vi "Extract_ROIs_miniScans.vi"(5 "ROI Attributes":T1[](array[typedef]) {"Apparent Frame Size" format="%#_6f"; "Original FOV (um)" format="%#_6f"; "Pixels per miniscan" format="%#_6f"; "Dwell Time per pixel" format="%#_6f"; "Resolution" format="%#_6f"; "ROI group ID" format="%#_6f"; "Laser Power (%)" format="%#_6f"; "Zoom" format="%#_6f"; "Frame Size" format="%#_6f"; "Number of lines" format="%#_6f"; "Composite ID" format="%#_6f"; "Angle (deg)" format="%#_6f"; "ROI Time (ns)" format="%#_6f"; "ROI ID" format="%#_6f"; "Pixels in ROI" format="%#_6f"; "ROI index" format="%#_6f"; "Z stop" format="%#_6f"; "Y stop" format="%#_6f"; "X stop" format="%#_6f"; "Z start" format="%#_6f"; "X start" format="%#_6f"; "Y start" format="%#_6f"}, 11 "error in (no error)":errorcluster) -> (1 "number of POI":i32, 3 "Number of pixels in single X miniscan":i32, 4 "ROI Coordinates (broken down to miniscans)":T2, 6 "miniScan_Indices":dbl[](array[numeric]), 8 "Total Pixels":i32, 10 "Total number of miniscans":i32, 12 "number of rectangles":i32, 13 "variable X Miniscan Pixels":i32[](array[numeric]), 14 "Zoom":dbl[](array[numeric]), 15 "error out":errorcluster)   [LabVIEW 2020]
uses:
  Typedefs/ROI XY coordinates cluster.ctl
  User Interface/Visualisation/Functional Imaging Viewer/Typedefs/ROI parameters data type.ctl
panel:
  out "POI_Indices":dbl[](array[numeric])
  # "PRE-ALLOCATED CLONE RE-ENTRANT"
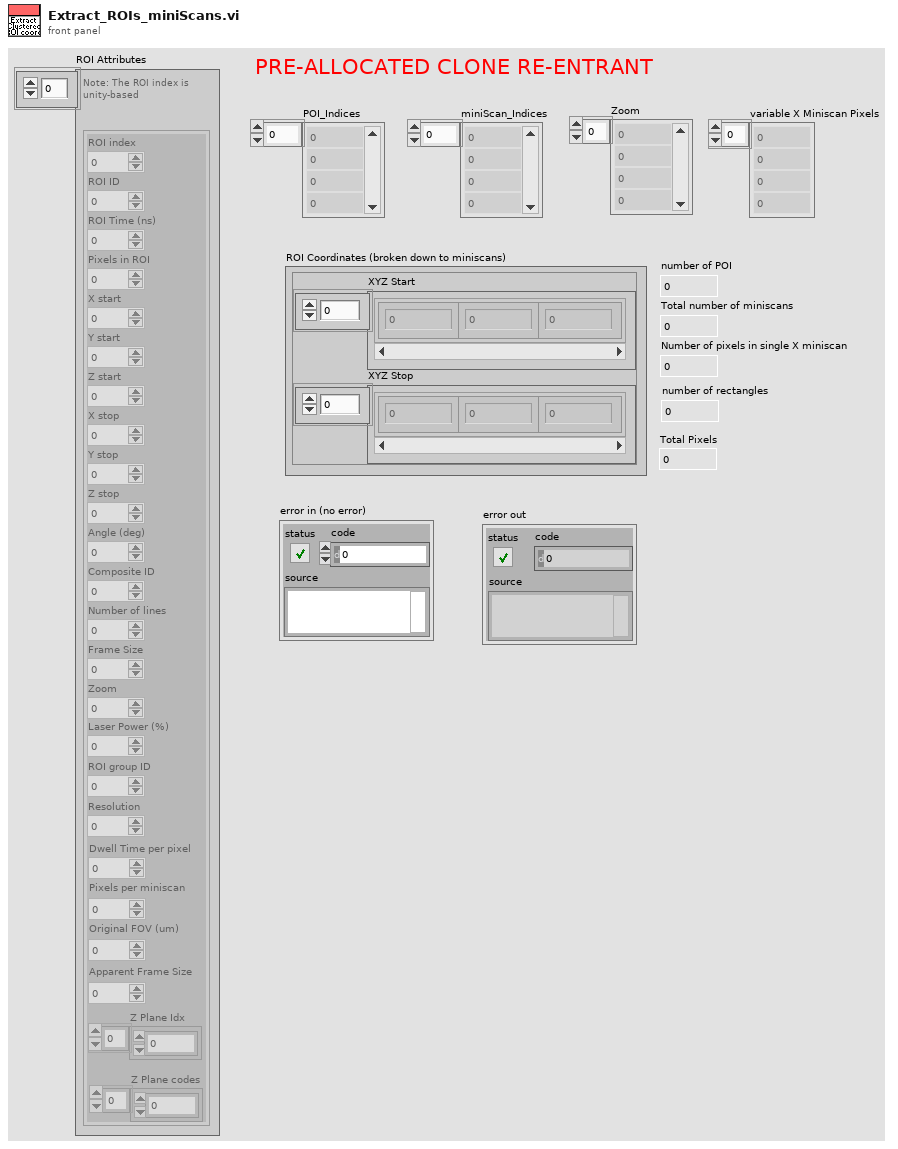
[diagram p1: front panel]
types:
  T1 = typedef "ROI parameters data type.ctl" = cluster{"ROI index":dbl, "ROI ID":dbl, "ROI Time (ns)":dbl, "Pixels in ROI":dbl, "X start":dbl, "Y start":dbl, "Z start":dbl, "X stop":dbl, "Y stop":dbl, "Z stop":dbl, "Angle (deg)":dbl, "Composite ID":dbl, "Number of lines":dbl, "Frame Size":dbl, "Zoom":dbl, "Laser Power (%)":dbl, "ROI group ID":dbl, "Resolution":dbl, "Dwell Time per pixel":dbl, "Pixels per miniscan":dbl, "Original FOV (um)":dbl, "Apparent Frame Size":dbl, "Z Plane Idx":i32[], "Z Plane codes":i32[]}
  T2 = typedef "ROI XY coordinates cluster.ctl" = cluster{"XYZ Start":cluster{"X":sgl, "Y":sgl, "Z":sgl}[], "XYZ Stop":cluster{"X":sgl, "Y":sgl, "Z":sgl}[]}
  T3 = cluster{"X start":dbl, "Y start":dbl, "Z start":dbl}[]
  T4 = cluster{"X start":dbl, "Y start":dbl, "Z start":dbl}
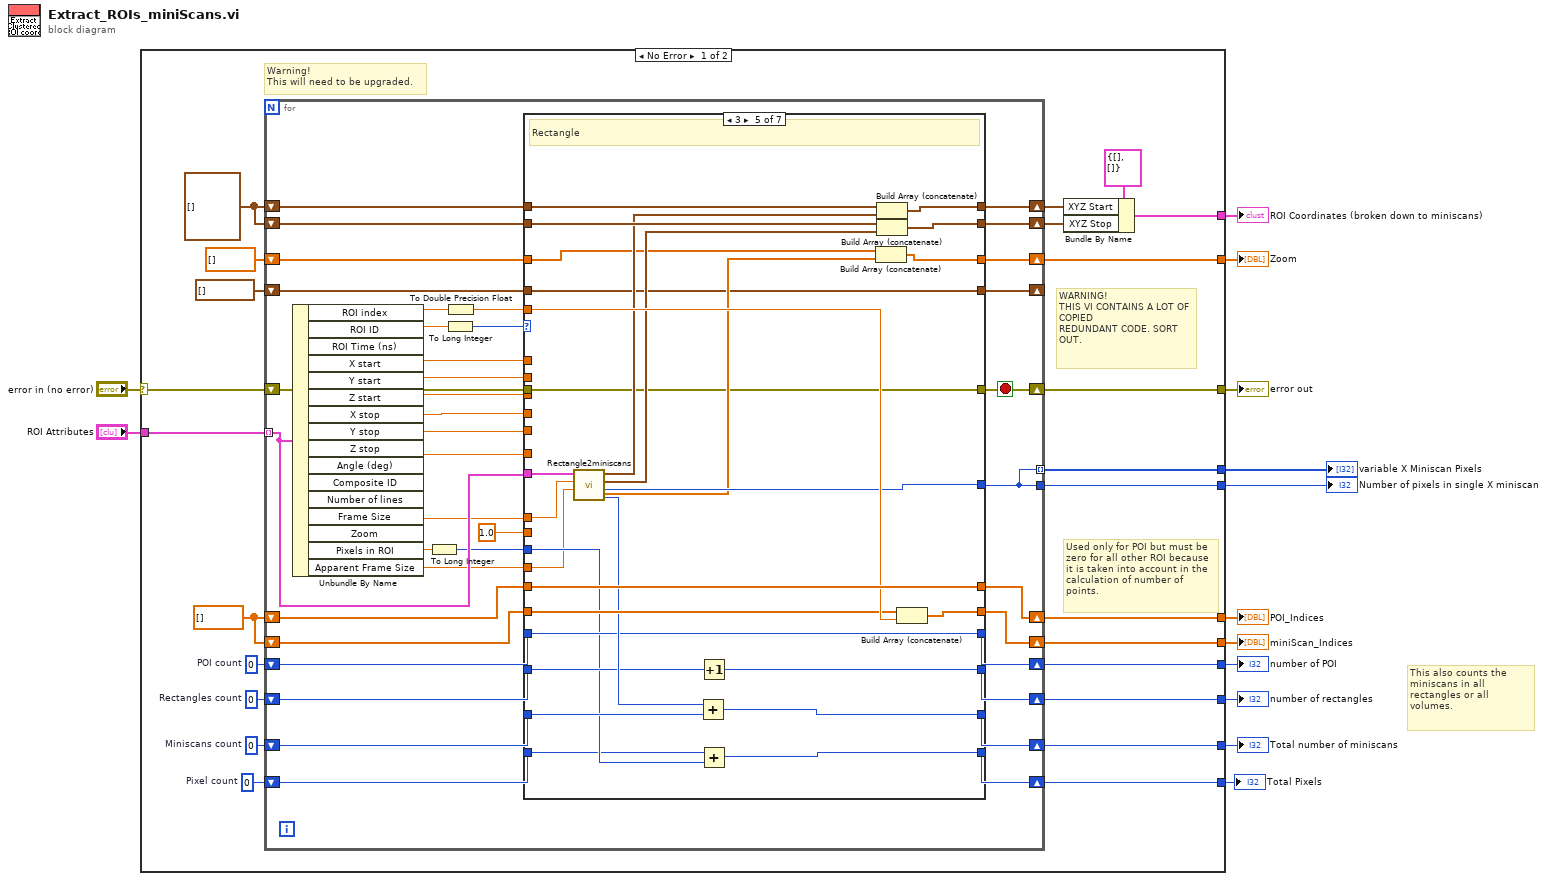
[diagram p0: block diagram]
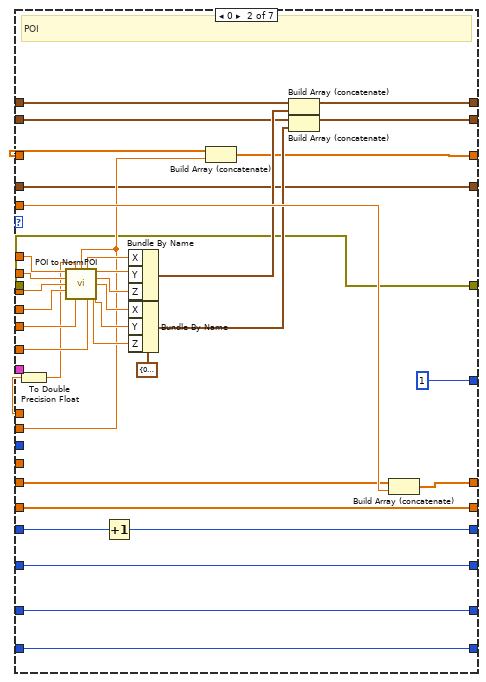
[diagram p3: hidden frame]
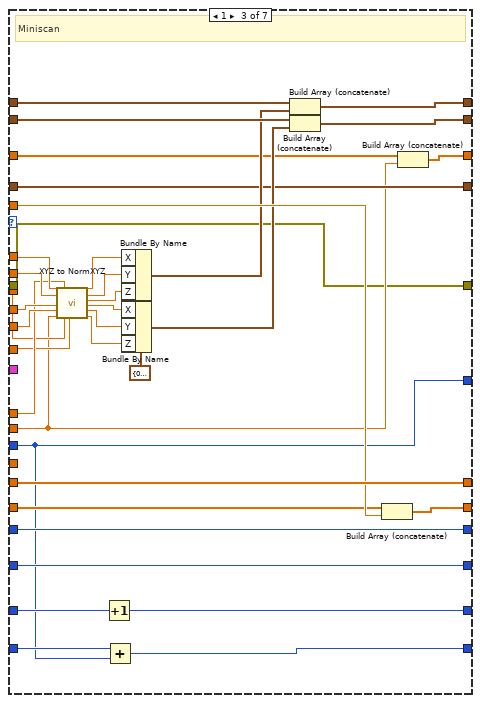
[diagram p4: hidden frame]
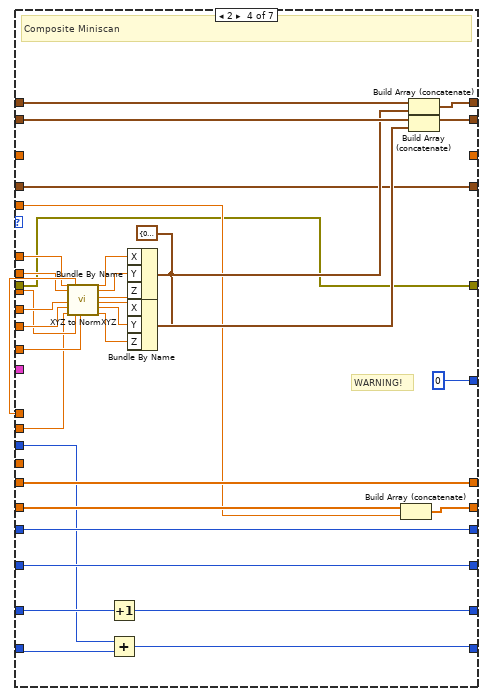
[diagram p5: hidden frame]
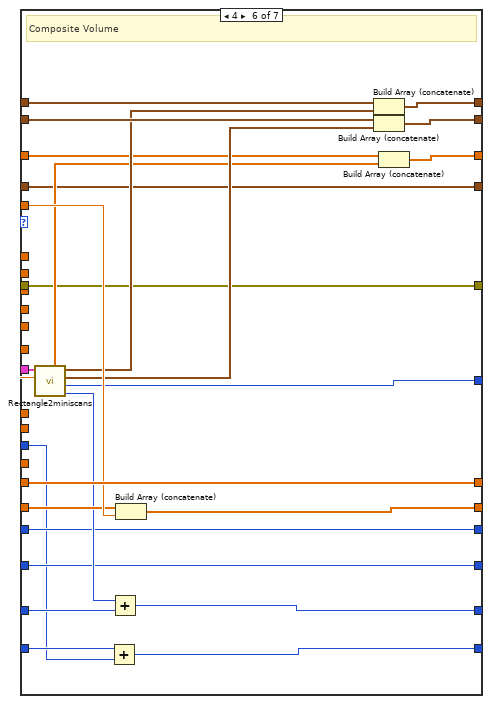
[diagram p6: hidden frame]
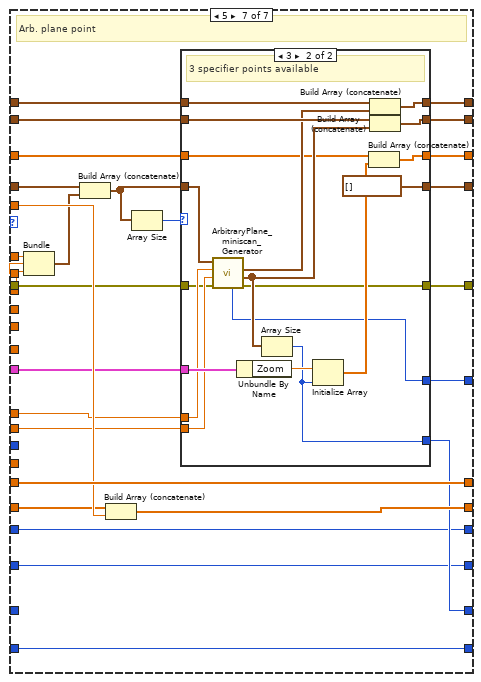
[diagram p7: hidden frame]
diagram:
  # "This also counts the miniscans in all rectangles or all volumes."
  n1 = case shown="No Error" "error in (no error)" {
    selector: "error in (no error)" -> [w20 w300]
    tunnel: [w19 w300] -> w12
    tunnel: [w28 _] -> w11
    tunnel: [w27 _] -> w10
    tunnel: [w26 _] -> w9
    tunnel: [w25 _] -> w8
    tunnel: [w24 _] -> w7
    tunnel: [w23 _] -> w6
    tunnel: [w22 _] -> w5
    tunnel: "ROI Attributes" -> [w21 _]
    tunnel: [w18 _] -> w3
    tunnel: [w15 _] -> w2
    tunnel: [w14 _] -> w1
    frame No Error {
      w16 = 0  # Pixel count
      w17 = 0  # Rectangles count
      w30 = 0  # POI count
      w31 = 0  # Miniscans count
      w36 = cluster{"X":sgl, "Y":sgl, "Z":sgl}[] [] ("XYZ Coordinates")
      w37 = dbl[] []
      # "Used only for POI but must be zero for all other ROI because it is taken into account in the calculation of number of points."
      # "WARNING!\nTHIS VI CONTAINS A LOT OF COPIED \nREDUNDANT CODE. SORT OUT."
      # "Warning!\nThis will need to be upgraded."
      n2 = for {
        tunnel: w21 -> [w64] mode=indexing
        shift-right: [w74] -> w25
        shift-left: w37 -> [w73]
        shift-right: [w72] -> w24
        shift-left: w37 -> [w71]
        shift-right: [w70] -> w35
        shift-left: w36 -> [w69]
        shift-right: [w68] -> w34
        shift-left: w36 -> [w67]
        tunnel: [w40] -> w26
        shift-right: [w57] -> w27
        shift-left: dbl[] [] -> [w56]
        shift-right: [w52] -> w22
        shift-left: w31 -> [w53]
        shift-right: [w50] -> w23
        shift-left: w30 -> [w51]
        shift-right: [w49] -> _
        shift-left: T3 [] -> [w48]
        shift-right: [w46] -> w19
        shift-left: w20 -> [w47]
        shift-right: [w44] -> w18
        shift-left: w17 -> [w45]
        shift-right: [w41] -> w15
        shift-left: w16 -> [w42]
        tunnel: [w40] -> w14 mode=indexing
        stop <- w46 stop-if-true
        n3 = Unbundle By Name(w64) -> ("ROI index"=w75:dbl, "ROI ID"=w76:dbl, "X start"=w63:dbl, "Y start"=w62:dbl, "Z start"=w61:dbl, "X stop"=w60:dbl, "Y stop"=w59:dbl, "Z stop"=w58:dbl, "Frame Size"=w38:dbl, "Pixels in ROI"=w55:dbl, "Apparent Frame Size"=w39:dbl)  [unwired: 5 out]
        n4 = To Long Integer(number=w55) -> (32bit integer=w54:i32)
        n5 = To Long Integer(number=w76) -> (32bit integer=w65:i32)
        n6 = To Double Precision Float(number=w75) -> (double precision float=w66:dbl)
        n7 = case shown="3" w65 {
          tunnel: w66 -> [_ w122 w157 w184 w220 w246 w274]
          tunnel: [w84 w121 w158 w193 w221 w247 w275] -> w74
          tunnel: w73 -> [w84 w120 w158 w193 w221 w247 w275]
          tunnel: [w83 w119 w156 w192 w219 w245 w273] -> w72
          tunnel: w71 -> [w83 w119 w155 w191 w218 w244 w272]
          tunnel: [w86 w98 w154 w190 w217 w243 w271] -> w70
          tunnel: w69 -> [w86 w91 w153 w189 w216 w242 w270]
          tunnel: [w85 w97 w152 w188 w215 w241 w269] -> w68
          tunnel: w67 -> [w85 w90 w151 w187 w214 w240 w268]
          tunnel: w64 -> [_ _ _ _ w213 w239 w256]
          tunnel: w38 -> [_ w115 w135 w183 w212 w236 w260]
          tunnel: [_ 1 ("No of Pixels") w124 0 ("No of Pixels in a single miniscan") w209 w235 w254] -> w40
          tunnel: w63 -> [_ w108 w139 w182 _ _ w265]
          tunnel: w62 -> [_ w107 w138 w181 _ _ w264]
          tunnel: w61 -> [_ w106 w132 w170 _ _ w263]
          tunnel: w60 -> [_ w105 w137 w180 _ _ _]
          tunnel: w59 -> [_ w104 w136 w179 _ _ _]
          tunnel: w58 -> [_ w103 w131 w169 _ _ _]
          tunnel: [_ w99 w147 _ w207 w233 w267] -> w57
          tunnel: w56 -> [_ w100 w146 _ w203 w232 w266]
          tunnel: [w78 w95 w126 w162 w198 w225 w249] -> w50
          tunnel: 1.0 ("Zoom") -> [_ w101 w129 w166 _ _ w253]
          tunnel: w54 -> [_ _ w124 w161 w197 w222 _]
          tunnel: w53 -> [w82 w94 w134 w172 w205 w230 _]
          tunnel: [w82 w94 w133 w171 w204 w229 w255] -> w52
          tunnel: w51 -> [w78 w93 w126 w162 w198 w225 w249]
          tunnel: [w81 w92 w130 w167 w202 w228 w259] -> w49
          tunnel: w48 -> [w81 w92 w130 w167 w202 w228 w261]
          tunnel: w47 -> [w80 w89 w128 w164 w201 w227 w252]
          tunnel: [w80 w89 w128 w164 w201 w227 w251] -> w46
          tunnel: w45 -> [w79 w88 w127 w163 w200 w226 w250]
          tunnel: [w79 w88 w127 w163 w199 w226 w250] -> w44
          tunnel: w42 -> [w77 w87 w125 w160 w196 w224 w248]
          tunnel: [w77 w87 w123 w159 w195 w223 w248] -> w41
          tunnel: w39 -> [_ _ _ _ w194 _ _]
          frame Default {
          }
          frame 0 {
            w118 = cluster{"X":dbl, "Y":dbl, "Z":dbl} {"X"=0.0, "Y"=0.0, "Z"=0.0} ("XYZ")
            # "POI"
            n8 = To Double Precision Float(number=w115) -> (double precision float=w102:dbl)
            n9 = call "POI to NormPOI.vi"("X start"=w108, "FrameSize"=w102, "Zoom"=w101, "Y start"=w107, "Z start"=w106, "X stop"=w105, "Y stop"=w104, "Z stop"=w103) -> ("Norm XStart"=w113:dbl, "Norm YStart"=w114:dbl, "Norm ZStart"=w112:dbl, "Norm XStop"=w111:dbl, "Norm YStop"=w110:dbl, "Norm ZStop"=w109:dbl)  [unwired: 2 in]
            n10 = Increment(x=w93) -> (x+1=w95:i32)
            n11 = Bundle By Name(cluster=w118, "X"=w113, "Y"=w114, "Z"=w112) -> (w117:cluster{"X":dbl, "Y":dbl, "Z":dbl})
            n12 = Bundle By Name(cluster=w118, "X"=w111, "Y"=w110, "Z"=w109) -> (w116:cluster{"X":dbl, "Y":dbl, "Z":dbl})
            n13 = Build Array (concatenate)(w100, w101) -> (w99:dbl[])
            n14 = Build Array (concatenate)(w91, w117) -> (w98:cluster{"X":dbl, "Y":dbl, "Z":dbl}[])
            n15 = Build Array (concatenate)(w90, w116) -> (w97:cluster{"X":dbl, "Y":dbl, "Z":dbl}[])
            n16 = Build Array (concatenate)(w120, w122) -> (w121:dbl[])
          }
          frame 1 {
            w150 = cluster{"X":dbl, "Y":dbl, "Z":dbl} {"X"=0.0, "Y"=0.0, "Z"=0.0} ("XYZ")
            # "Miniscan"
            n17 = call "XYZ to NormXYZ.vi"("X start"=w139, "Y start"=w138, "X stop"=w137, "Y stop"=w136, "Zoom (either ref or main zoom)"=w129, "FrameSize"=w135, "Z start"=w132, "Z stop"=w131) -> ("Norm X Start"=w145:dbl, "Norm Y Start"=w144:dbl, "Norm Z Start"=w143:dbl, "Norm X Stop"=w142:dbl, "Norm Y Stop"=w141:dbl, "Norm Z Stop"=w140:dbl)  [unwired: 6 in]
            n18 = Increment(x=w134) -> (x+1=w133:i32)
            n19 = Add(x=w125, y=w124) -> (x+y=w123:i32)
            n20 = Bundle By Name(cluster=w150, "X"=w145, "Y"=w144, "Z"=w143) -> (w149:cluster{"X":dbl, "Y":dbl, "Z":dbl})
            n21 = Bundle By Name(cluster=w150, "X"=w142, "Y"=w141, "Z"=w140) -> (w148:cluster{"X":dbl, "Y":dbl, "Z":dbl})
            n22 = Build Array (concatenate)(w153, w149) -> (w154:cluster{"X":dbl, "Y":dbl, "Z":dbl}[])
            n23 = Build Array (concatenate)(w151, w148) -> (w152:cluster{"X":dbl, "Y":dbl, "Z":dbl}[])
            n24 = Build Array (concatenate)(w155, w157) -> (w156:dbl[])
            n25 = Build Array (concatenate)(w146, w129) -> (w147:dbl[])
          }
          frame 2 {
            w165 = cluster{"X":dbl, "Y":dbl, "Z":dbl} {"X"=0.0, "Y"=0.0, "Z"=0.0} ("XYZ")
            # "WARNING!"
            # "Composite Miniscan"
            n26 = call "XYZ to NormXYZ.vi"("X start"=w182, "Y start"=w181, "X stop"=w180, "Y stop"=w179, "Zoom (either ref or main zoom)"=w166, "FrameSize"=w183, "Z start"=w170, "Z stop"=w169) -> ("Norm X Start"=w178:dbl, "Norm Y Start"=w177:dbl, "Norm Z Start"=w176:dbl, "Norm X Stop"=w175:dbl, "Norm Y Stop"=w174:dbl, "Norm Z Stop"=w173:dbl)  [unwired: 6 in]
            n27 = Increment(x=w172) -> (x+1=w171:i32)
            n28 = Add(x=w161, y=w160) -> (x+y=w159:i32)
            n29 = Bundle By Name(cluster=w165, "X"=w178, "Y"=w177, "Z"=w176) -> (w186:cluster{"X":dbl, "Y":dbl, "Z":dbl})
            n30 = Bundle By Name(cluster=w165, "X"=w175, "Y"=w174, "Z"=w173) -> (w185:cluster{"X":dbl, "Y":dbl, "Z":dbl})
            n31 = Build Array (concatenate)(w191, w184) -> (w192:dbl[])
            n32 = Build Array (concatenate)(w189, w186) -> (w190:cluster{"X":dbl, "Y":dbl, "Z":dbl}[])
            n33 = Build Array (concatenate)(w187, w185) -> (w188:cluster{"X":dbl, "Y":dbl, "Z":dbl}[])
          }
          frame 3 {
            # "Rectangle"
            n34 = call "Rectangle2miniscans.vi"("Apparent Frame Size"=w194, "Frame Size"=w212, "X-Y-Z coordinates"=w213) -> ("No of Miniscans"=w206:i32, "No of Pixels in a single miniscan"=w209:i32, "XYZ Stop"=w210:cluster{"X":dbl, "Y":dbl, "Z":dbl}[], "XYZ Start"=w211:cluster{"X":dbl, "Y":dbl, "Z":dbl}[], "Zoom"=w208:dbl[])  [unwired: 4 in]
            n35 = Add(x=w206, y=w205) -> (x+y=w204:i32)
            n36 = Increment(x=w200) -> (x+1=w199:i32)
            n37 = Add(x=w196, y=w197) -> (x+y=w195:i32)
            n38 = Build Array (concatenate)(w203, w208) -> (w207:dbl[])
            n39 = Build Array (concatenate)(w216, w211) -> (w217:cluster{"X":dbl, "Y":dbl, "Z":dbl}[])
            n40 = Build Array (concatenate)(w214, w210) -> (w215:cluster{"X":dbl, "Y":dbl, "Z":dbl}[])
            n41 = Build Array (concatenate)(w218, w220) -> (w219:dbl[])
          }
          frame 4 {
            # "Composite Volume"
            n42 = call "Rectangle2miniscans.vi"("Frame Size"=w236, "X-Y-Z coordinates"=w239) -> ("No of Miniscans"=w231:i32, "No of Pixels in a single miniscan"=w235:i32, "XYZ Stop"=w237:cluster{"X":dbl, "Y":dbl, "Z":dbl}[], "XYZ Start"=w238:cluster{"X":dbl, "Y":dbl, "Z":dbl}[], "Zoom"=w234:dbl[])  [unwired: 5 in]
            n43 = Add(x=w224, y=w222) -> (x+y=w223:i32)
            n44 = Add(x=w231, y=w230) -> (x+y=w229:i32)
            n45 = Build Array (concatenate)(w244, w246) -> (w245:dbl[])
            n46 = Build Array (concatenate)(w242, w238) -> (w243:cluster{"X":dbl, "Y":dbl, "Z":dbl}[])
            n47 = Build Array (concatenate)(w240, w237) -> (w241:cluster{"X":dbl, "Y":dbl, "Z":dbl}[])
            n48 = Build Array (concatenate)(w232, w234) -> (w233:dbl[])
          }
          frame 5 {
            # "Arb. plane point"
            n49 = Bundle("X start"=w265, "Y start"=w264, "Z start"=w263) -> (w262:T4)  [unwired: 1 in]
            n50 = Build Array (concatenate)(w261, w262) -> (w258:T3)
            n51 = Build Array (concatenate)(w272, w274) -> (w273:dbl[])
            n52 = Array Size(array=w258) -> (size(s)=w257:i32)
            n53 = case shown="3" w257 {
              tunnel: [w279 w299] -> w271
              tunnel: w270 -> [w279 w298]
              tunnel: [w278 w297] -> w269
              tunnel: w268 -> [w278 w296]
              tunnel: [w277 w295] -> w267
              tunnel: w266 -> [w277 w286]
              tunnel: w258 -> [w280 w294]
              tunnel: w260 -> [_ w285]
              tunnel: [w280 T3 []] -> w259
              tunnel: w256 -> [_ w291]
              tunnel: [_ w287] -> w255
              tunnel: [_ w282] -> w254
              tunnel: w253 -> [_ w284]
              tunnel: w252 -> [w276 w283]
              tunnel: [w276 w281] -> w251
              frame Default {
                # "< than 3 specifier points"
              }
              frame 3 {
                # "3 specifier points available"
                n54 = call "ArbitraryPlane_miniscan_Generator.vi"("error in"=w283, "Main Zoom"=w284, "Frame Size"=w285, "Input data"=w294) -> ("error out"=w281:errorcluster, "XYZ Stop Norm"=w290:cluster{"X":sgl, "Y":sgl, "Z":sgl}[], "XYZ Start Norm"=w292:cluster{"X":sgl, "Y":sgl, "Z":sgl}[], "Number of pixels in single X miniscan"=w282:i32)  [unwired: 3 in, 1 out]
                n55 = Unbundle By Name(w291) -> ("Zoom"=w289:dbl)
                n56 = Array Size(array=w290) -> (size(s)=w287:i32)
                n57 = Initialize Array(w289, w287) -> (w288:dbl[])
                n58 = Build Array (concatenate)(w286, w288) -> (w295:dbl[])
                n59 = Build Array (concatenate)(w298, w292) -> (w299:cluster{"X":dbl, "Y":dbl, "Z":dbl}[])
                n60 = Build Array (concatenate)(w296, w290) -> (w297:cluster{"X":dbl, "Y":dbl, "Z":dbl}[])
              }
            }
          }
        }
      }
      n61 = Bundle By Name(cluster=T2 {"XYZ Start"=[], "XYZ Stop"=[]} ("ROI Coordinates"), "XYZ Start"=w35, "XYZ Stop"=w34) -> (w28:T2)
    }
    frame Error {
    }
  }
  "error out" <- w12
  "ROI Coordinates (broken down to miniscans)" <- w11
  "POI_Indices" <- w8
  "miniScan_Indices" <- w7
  "Total number of miniscans" <- w5
  "Number of pixels in single X miniscan" <- w9
  "Zoom" <- w10
  "number of POI" <- w6
  "number of rectangles" <- w3
  "Total Pixels" <- w2
  "variable X Miniscan Pixels" <- w1
